vi "(SubVI)System Command_Firmware Update.vi"(7 "popup":bool, 8 "error in (no error)":errorcluster caption="에러 입력(에러 없음)", 11 "FW File":path) -> (0 "error out":errorcluster caption="에러 출력", 3 "BD Info Str":string)   [LabVIEW 2020]
uses:
  Serial/Controls/(Ctrl)Serial_Write Read Option.ctl
  <vilib>/Utility/miscctls.llb/LVPointTypeDef.ctl
  43a18d0d-6580-4b88-920a-edf357bf0f71.vi
  Variables/(Var)System Variables.vi
panel:
  out "Slide":u8(slide) scale=0.0..4.0
  out "Status":string
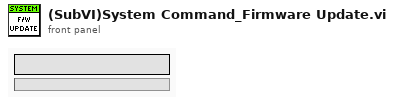
[diagram p1: front panel]
types:
  T1 = typedef "LVPointTypeDef.ctl" = cluster{"Horizontal":i16, "Vertical":i16}
  T2 = typedef "(Ctrl)Serial_Write Read Option.ctl" = cluster{"Echo Request":bool, "Header Verification":bool, "Checksum Verification":bool, "User Code Verifiaction":bool}
  T3 = enum32{"Invalid", "Standard", "Closed", "Hidden", "Minimized", "Maximized"}
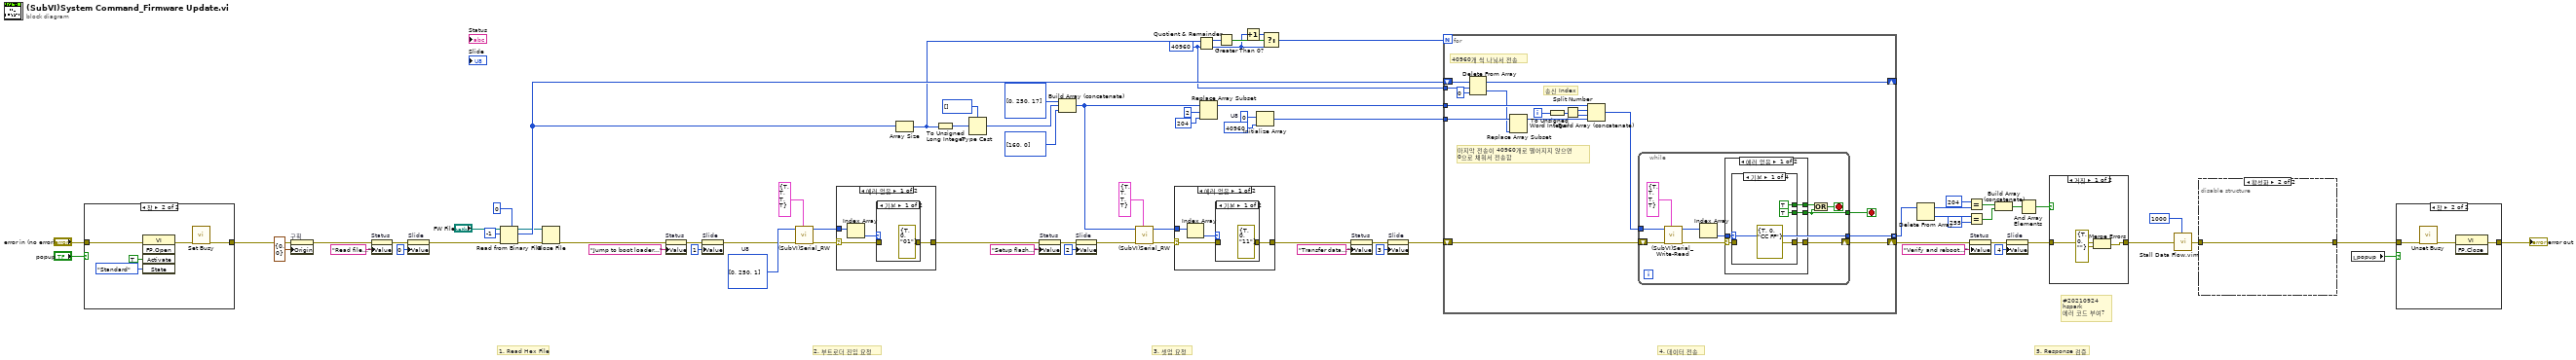
[diagram p0: block diagram]
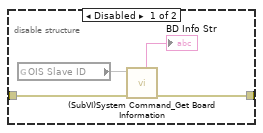
[diagram p3: hidden frame]
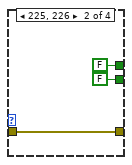
[diagram p9: hidden frame]
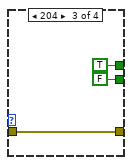
[diagram p10: hidden frame]
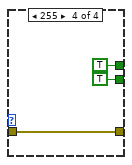
[diagram p11: hidden frame]
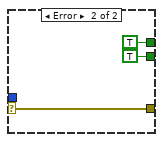
[diagram p12: hidden frame]
diagram:
  w39 = u8[] [0, 250, 1]  # U8
  w59 = u8 0  # U8
  w65 = 40960 ("y")
  # "5. Response 검증"
  # "4. 데이터 전송"
  # "3. 셋업 요청"
  # "2. 부트로더 진입 요청"
  # "1. Read Hex File"
  # "#20210924\nhspark\n에러 코드 부여?"
  n1 = case shown="참" "popup" {
    tunnel: "error in (no error)" -> [w77 w80]
    tunnel: [w77 w78] -> w2
    frame False {
    }
    frame True {
      n2 = invoke class="VI" method="FP.Open"(error in=w80, "Activate"=TRUE ("활성화?"), "State"=T3."Standard" ("상태")) -> (error out=w79:errorcluster)  [unwired: 2 in, 4 out]
      n3 = call <vilib>:"Set Busy.vi"("error in (no error)"=w79) -> ("error out"=w78:errorcluster)  [unwired: 9 in, 1 out]
    }
  }
  n4 = property on="구획" class="Pane"(error in=w2, "Origin"=T1 {"Horizontal"=0, "Vertical"=0} ("원점")) -> (error out=w34:errorcluster)  [unwired: 1 in, 1 out]
  n5 = property on="Status" class="Str"(error in=w34, "Value"="Read file..." ("Status")) -> (error out=w33:errorcluster)  [unwired: 1 in, 1 out]
  n6 = property on="Slide" class="Slide (엄격한)"(error in=w33, "Value"=u8 0 ("Slide")) -> (error out=w30:errorcluster)  [unwired: 1 in, 1 out]
  n7 = Read from Binary File(5:u8 0, 8:w30, 10:-1 ("카운트(1)"), 11:"FW File") -> (0:w63:errorcluster, 2:w69:u8[], 3:w64:refnum<file>)  [unwired: 2 in, 1 out]
  n8 = Close File(refnum=w64, error in=w63) -> (error out=w26:errorcluster)  [unwired: 1 out]
  n9 = property on="Status" class="Str"(error in=w26, "Value"="Jump to boot loader..." ("Status")) -> (error out=w27:errorcluster)  [unwired: 1 in, 1 out]
  n10 = property on="Slide" class="Slide (엄격한)"(error in=w27, "Value"=u8 1 ("Slide")) -> (error out=w25:errorcluster)  [unwired: 1 in, 1 out]
  n11 = call-poly "(SubVI)Serial_RW.vi"("Option"=T2 {"Echo Request"=TRUE, "Header Verification"=TRUE, "Checksum Verification"=TRUE, "User Code Verifiaction"=TRUE}, "error in (no error)"=w25, "Data to Write"=w39) -> ("error out"=w48:errorcluster, "Read Data"=w49:u8[])  [unwired: 6 in, 1 out]
  n12 = case shown="에러 없음" w48 {
    selector: w48 -> [w85 w89]
    tunnel: w49 -> [w86 _]
    tunnel: [w84 w89] -> w8
    frame No Error {
      n13 = Index Array(array=w86) -> (element=w83:u8)  [unwired: 1 in]
      n14 = case shown="기본" w83 {
        tunnel: w85 -> [_ w88]
        tunnel: [errorcluster {"status"=TRUE, "code"=0, "source"="01"} ("error IO") w88] -> w84
        frame Default {
        }
        frame 1 {
        }
      }
    }
    frame Error {
    }
  }
  n15 = Array Size(array=w69) -> (size(s)=w68:i32)
  n16 = To Unsigned Long Integer(number=w68) -> (unsigned 32bit integer=w67:u32)
  n17 = Type Cast(type=u8[] [], x=w67) -> (*(type *) &x=w50:u8[])
  n18 = property on="Status" class="Str"(error in=w8, "Value"="Setup flash..." ("Status")) -> (error out=w24:errorcluster)  [unwired: 1 in, 1 out]
  n19 = Build Array (concatenate)(u8[] [0, 250, 17] ("User Code"), w50, u8[] [160, 0] ("User Code")) -> (w38:u8[])
  n20 = property on="Slide" class="Slide (엄격한)"(error in=w24, "Value"=u8 2 ("Slide")) -> (error out=w7:errorcluster)  [unwired: 1 in, 1 out]
  n21 = call-poly "(SubVI)Serial_RW.vi"("Option"=T2 {"Echo Request"=TRUE, "Header Verification"=TRUE, "Checksum Verification"=TRUE, "User Code Verifiaction"=TRUE}, "error in (no error)"=w7, "Data to Write"=w38) -> ("error out"=w61:errorcluster, "Read Data"=w60:u8[])  [unwired: 6 in, 1 out]
  n22 = case shown="에러 없음" w61 {
    selector: w61 -> [w93 w96]
    tunnel: w60 -> [w91 _]
    tunnel: [w92 w96] -> w18
    frame No Error {
      n23 = Index Array(array=w91) -> (element=w90:u8)  [unwired: 1 in]
      n24 = case shown="기본" w90 {
        tunnel: w93 -> [_ w95]
        tunnel: [errorcluster {"status"=TRUE, "code"=0, "source"="11"} ("error IO") w95] -> w92
        frame Default {
        }
        frame 17 {
        }
      }
    }
    frame Error {
    }
  }
  n25 = Quotient & Remainder(x=w68, y=w65) -> (x-y*floor(x/y)=w74:i32, floor(x/y)=w72:i32)
  n26 = Replace Array Subset(array=w38, new element=u8 204 ("User Code"), index=2 ("인덱스")) -> (w55:u8[])
  n27 = Greater Than 0?(x=w74) -> (x > 0?=w73:bool)
  n28 = Increment(x=w72) -> (x+1=w71:i32)
  n29 = Initialize Array(w59, 40960 ("차원 크기")) -> (w54:u8[])
  n30 = Select(t=w71, s=w73, f=w72) -> (s? t:f=w70:i32)
  n31 = property on="Status" class="Str"(error in=w18, "Value"="Transfer data..." ("Status")) -> (error out=w19:errorcluster)  [unwired: 1 in, 1 out]
  n32 = property on="Slide" class="Slide (엄격한)"(error in=w19, "Value"=u8 3 ("Slide")) -> (error out=w10:errorcluster)  [unwired: 1 in, 1 out]
  n33 = for {
    N: w70 -> [_]
    tunnel: w65 -> [w112]
    shift-right: [w111] -> _
    shift-left: w69 -> [w113]
    shift-right: [w101] -> w9
    shift-left: w10 -> [w108]
    tunnel: [w110] -> w46 mode=indexing
    tunnel: w55 -> [w109]
    tunnel: w54 -> [w104]
    i -> [w98]
    stop <- w100 stop-if-true
    # "40960개 씩 나눠서 전송"
    # "마지막 전송이 40960개로 떨어지지 않으면\n0으로 채워서 전송함"
    # "송신 Index"
    n34 = Delete From Array(array=w113, length=w112, index=0 ("인덱스")) -> (deleted portion=w103:u8[], array with subset deleted=w111:u8[])
    n35 = Replace Array Subset(array=w104, new element=w103) -> (w102:u8[])  [unwired: 1 in]
    n36 = To Unsigned Word Integer(number=w98) -> (unsigned 16bit integer=w107:u16)
    n37 = Split Number(x=w107) -> (hi(x)=w106:u8, lo(x)=w105:u8)
    n38 = Build Array (concatenate)(w109, w106, w105, w102) -> (w97:u8[])
    n39 = while {
      shift-right: [w118] -> w101
      shift-left: w108 -> [w122]
      tunnel: w97 -> [w121]
      tunnel: [w114] -> w110
      tunnel: [w115] -> w100
      stop <- w116 stop-if-true
      n40 = call "(SubVI)Serial_Write-Read.vi"("Option"=T2 {"Echo Request"=TRUE, "Header Verification"=TRUE, "Checksum Verification"=TRUE, "User Code Verifiaction"=TRUE}, "error in (no error)"=w122, "Data to Write"=w121) -> ("error out"=w119:errorcluster, "Read Data"=w123:u8[])  [unwired: 6 in, 1 out]
      n41 = Index Array(array=w123) -> (element=w114:u8)  [unwired: 1 in]
      n42 = case shown="에러 없음" w119 {
        selector: w119 -> [w126 w143]
        tunnel: w114 -> [w128 _]
        tunnel: [w127 TRUE] -> w117
        tunnel: [w125 w143] -> w118
        tunnel: [w124 TRUE] -> w115
        frame No Error {
          n43 = case shown="기본" w128 {
            tunnel: [TRUE FALSE TRUE TRUE] -> w127
            tunnel: w126 -> [_ w133 w136 w139]
            tunnel: [errorcluster {"status"=TRUE, "code"=0, "source"="CC FF"} ("에러 입력") w133 w136 w139] -> w125
            tunnel: [TRUE FALSE FALSE TRUE] -> w124
            frame Default {
            }
            frame 225, 226 {
            }
            frame 204 {
            }
            frame 255 {
            }
          }
        }
        frame Error {
        }
      }
      n44 = Or(x=w117, y=w115) -> (x .or. y?=w116:bool)
    }
  }
  n45 = Delete From Array(array=w46) -> (deleted portion=w45:u8, array with subset deleted=w44:u8[])  [unwired: 2 in]
  n46 = Equal?(x=u8 204, y=w44) -> (x = y?=w43:bool[])
  n47 = Equal?(x=w45, y=u8 255) -> (x = y?=w42:bool)
  n48 = property on="Status" class="Str"(error in=w9, "Value"="Verify and reboot..." ("Status")) -> (error out=w17:errorcluster)  [unwired: 1 in, 1 out]
  n49 = Build Array (concatenate)(w43, w42) -> (w41:bool[])
  n50 = property on="Slide" class="Slide (엄격한)"(error in=w17, "Value"=u8 4 ("Slide")) -> (error out=w14:errorcluster)  [unwired: 1 in, 1 out]
  n51 = And Array Elements(Boolean array=w41) -> (logical AND=w40:bool)
  n52 = case shown="거짓" w40 {
    tunnel: w14 -> [w146 w147]
    tunnel: [w145 w147] -> w13
    frame False {
      n53 = Merge Errors(w146, errorcluster {"status"=TRUE, "code"=0, "source"=""} ("에러 입력")) -> (w145:errorcluster)
    }
    frame True {
    }
  }
  n54 = call "Stall Data Flow.vim"("value in"=w13, "milliseconds to wait"=u32 1000) -> ("value out"=w12:errorcluster)  [unwired: 1 out]
  n55 = disable-structure shown="활성화" {
    disable-tunnel: w12 -> [w151 w152]
    disable-tunnel: [w148 w152] -> w1
    frame Disabled {
      n56 = global read "(Var)System Variables.vi" "OIS Slave ID"() -> (w150)
      n57 = call "(SubVI)System Command_Get Board Information.vi"("error in (no error)"=w151, "ID to Find"=w150) -> ("error out"=w148:errorcluster, "BD SN"=→"BD Info Str":string)  [unwired: 2 in, 6 out]
    }
    frame Enabled {
    }
  }
  n58 = local read "popup"() -> (w4:bool)
  n59 = case shown="참" w4 {
    tunnel: w1 -> [w153 w156]
    tunnel: [w153 w155] -> w3
    frame False {
    }
    frame True {
      n60 = call <vilib>:"Unset Busy.vi"("error in (no error)"=w156) -> ("error out"=w154:errorcluster)  [unwired: 10 in]
      n61 = invoke class="VI" method="FP.Close"(error in=w154) -> (error out=w155:errorcluster)  [unwired: 2 in, 2 out]
    }
  }
  "error out" <- w3
